vi "AprilTagPoseEstimate_GetAmbifuity.vi"(11 "AprilTagPoseEstimate":T1={"AprilTransform3d_1"={"TRANSLATION3D"={"X"=0.0, "Y"=0.0, "Z"=0.0}, "ROTATION3D"={"Q_quaternion"={"R"=1.0, "V"=[0.0, 0.0, 0.0]}}, "XF"=FALSE}, "AprilTransform3d_2"={"TRANSLATION3D"={"X"=0.0, "Y"=0.0, "Z"=0.0}, "ROTATION3D"={"Q_quaternion"={"R"=1.0, "V"=[0.0, 0.0, 0.0]}}, "XF"=FALSE}, "Error1"=0.0, "Error2"=0.0} {"AprilTransform3d_2"."TRANSLATION3D"."Z" format="%14.3f"; "AprilTransform3d_2"."TRANSLATION3D"."Y" format="%14.3f"; "AprilTransform3d_2"."TRANSLATION3D"."X" format="%14.3f"; "AprilTransform3d_1"."TRANSLATION3D"."Z" format="%14.3f"; "AprilTransform3d_1"."TRANSLATION3D"."Y" format="%14.3f"; "AprilTransform3d_1"."TRANSLATION3D"."X" format="%14.3f"}) -> (3 "Ambiguity":dbl)   [LabVIEW 2019, in "Trajectory_Library.lvlib"]
uses:
  TypeDef/TRANSLATION3D.ctl
  TypeDef/ROTATION3D.ctl
  TypeDef/QUATERNION.ctl
  Trajectory_Library.lvlib
  TypeDef/TRANSFORM3D.ctl
  TypeDef/AprilTagPoseEstimate.ctl
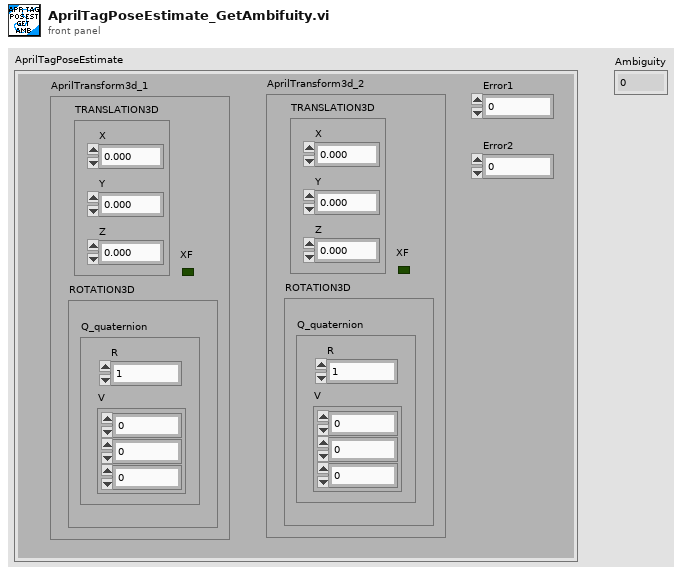
[diagram p1: front panel]
types:
  T1 = typedef "Trajectory_Library.lvlib/AprilTagPoseEstimate.ctl" = cluster{"AprilTransform3d_1":T2, "AprilTransform3d_2":T2, "Error1":dbl, "Error2":dbl}
  T2 = typedef "Trajectory_Library.lvlib/TRANSFORM3D.ctl" = cluster{"TRANSLATION3D":T3, "ROTATION3D":T4, "XF":bool}
  T3 = typedef "Trajectory_Library.lvlib/TRANSLATION3D.ctl" = cluster{"X":dbl, "Y":dbl, "Z":dbl}
  T4 = typedef "Trajectory_Library.lvlib/ROTATION3D.ctl" = cluster{"Q_quaternion":T5}
  T5 = typedef "Trajectory_Library.lvlib/QUATERNION.ctl" = cluster{"R":dbl, "V":dbl[]}
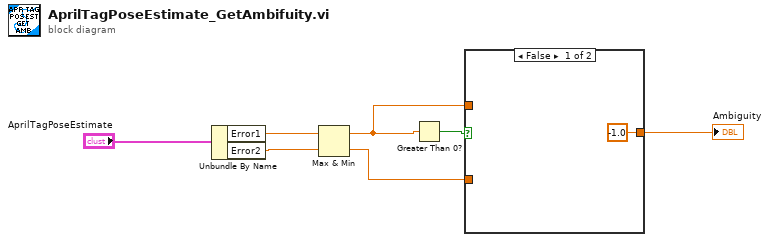
[diagram p0: block diagram]
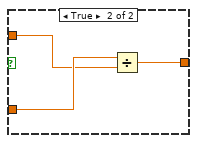
[diagram p2: hidden frame]
diagram:
  n1 = Unbundle By Name("AprilTagPoseEstimate") -> ("Error1"=w6:dbl, "Error2"=w5:dbl)
  n2 = Max & Min(x=w6, y=w5) -> (max(x,y)=w3:dbl, min(x,y)=w2:dbl)
  n3 = Greater Than 0?(x=w3) -> (x > 0?=w4:bool)
  n4 = case shown="False" w4 {
    tunnel: w3 -> [_ w10]
    tunnel: w2 -> [_ w11]
    tunnel: [-1.0 w9] -> w1
    frame False {
    }
    frame True {
      n5 = Divide(x=w11, y=w10) -> (x/y=w9:dbl)
    }
  }
  "Ambiguity" <- w1
